vi "smartmeshIP serial mux init.vi"(8 "error in (no error)":errorcluster, 11 "serial mux adress":T1={"serial_mux IP"="127.0.0.1", "rserial_mux port"=9900}) -> (0 "error out":errorcluster, 3 "connection ID out":refnum<k5>)   [LabVIEW 2017]
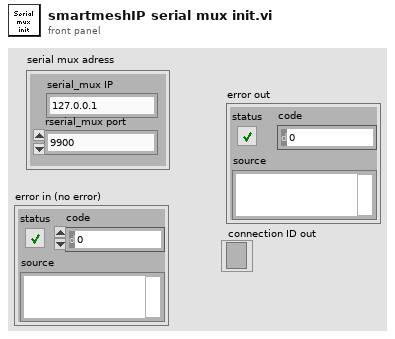
[diagram p1: front panel]
types:
  T1 = cluster{"serial_mux IP":string, "rserial_mux port":u16}
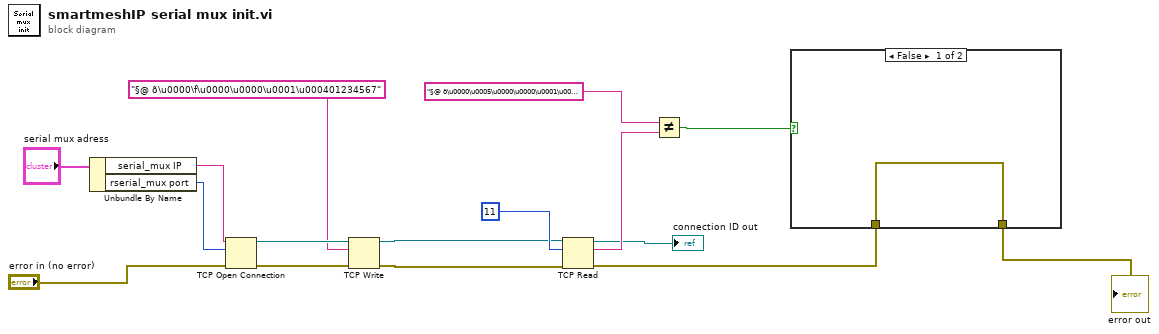
[diagram p0: block diagram]
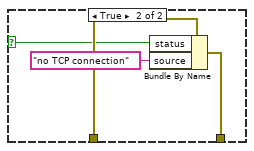
[diagram p2: hidden frame]
diagram:
  n1 = Unbundle By Name("serial mux adress") -> ("serial_mux IP"=w5:string, "rserial_mux port"=w4:u16)
  n2 = TCP Open Connection(address=w5, remote port or service name=w4, error in (no error)="error in (no error)") -> (connection ID=w15:refnum<k5>, error out=w16:errorcluster)  [unwired: 2 in]
  n3 = TCP Write(connection ID=w15, data in="§@ õ\u0000\f\u0000\u0000\u0001\u000401234567", error in (no error)=w16) -> (connection ID out=w13:refnum<k5>, error out=w12:errorcluster)  [unwired: 1 in, 1 out]
  n4 = TCP Read(connection ID=w13, bytes to read=11, error in (no error)=w12) -> (connection ID out=→"connection ID out":refnum<k5>, data out=w9:string, error out=w7:errorcluster)  [unwired: 2 in]
  n5 = Not Equal?(x="§@ õ\u0000\u0005\u0000\u0000\u0001\u0000\u0004" ("data in"), y=w9) -> (x != y?=w8:bool)
  n6 = case shown="False" w8 {
    selector: w8 -> [_ w19]
    tunnel: w7 -> [w17 w21]
    tunnel: [w17 w20] -> w3
    frame False {
    }
    frame True {
      n7 = Bundle By Name(cluster=w21, "status"=w19, "source"="no TCP connection") -> (w20:errorcluster)
    }
  }
  "error out" <- w3
